vi "Filter File Names by Extension.vi"(8 "Error In":errorcluster, 9 "patterns":string, 11 "filenames in":string[](array[string])) -> (0 "Error Out":errorcluster, 1 "# Discarded":i32, 3 "filenames out":string[](array[string]))   [LabVIEW 2021, in "Files.lvlib"]
uses:
  Files.lvlib
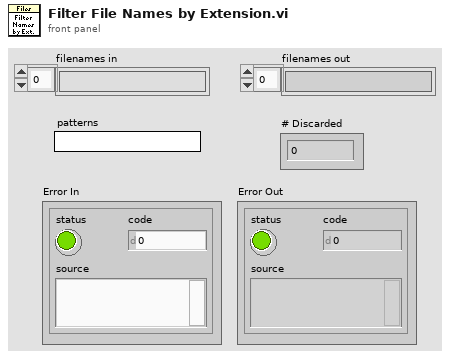
[diagram p1: front panel]
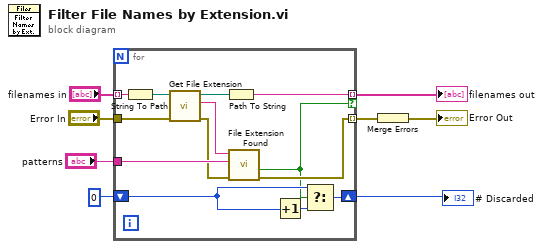
[diagram p0: block diagram]
diagram:
  n1 = for {
    tunnel: "filenames in" -> [w21] mode=indexing
    tunnel: "Error In" -> [w19]
    tunnel: [w13] -> w6 mode=indexing
    tunnel: [w17] -> w3 mode=indexing if=w9
    tunnel: "patterns" -> [w15]
    shift-right: [w12] -> w1
    shift-left: 0 -> [w10]
    n2 = String To Path(string=w21) -> (path=w20:path)
    n3 = call <vilib>:"Get File Extension.vi"("error in (no error)"=w19, "file"=w20) -> ("error out"=w14:errorcluster, "lowercase file extension"=w16:string, "dup file"=w18:path)  [unwired: 5 in, 2 out]
    n4 = Path To String(path=w18) -> (string=w17:string)
    n5 = call "File Extension Found.vi"("error in (no error)"=w14, "patterns"=w15, "lowercase file extension"=w16) -> ("error out"=w13:errorcluster, "match?"=w9:bool)  [unwired: 5 in, 2 out]
    n6 = Increment(x=w10) -> (x+1=w11:i32)
    n7 = Select(t=w10, s=w9, f=w11) -> (s? t:f=w12:i32)
  }
  "filenames out" <- w3
  "# Discarded" <- w1
  n8 = Merge Errors(w6) -> (→"Error Out":errorcluster)
